vi "App.vi"() -> ()   [LabVIEW 2023]
uses:
  <vilib>/Instr/_visa.llb/VISA Configure Serial Port (Instr).vi
panel:
  out "Waveform Chart":dbl(graph)
  out "Temperatura Actual":string
  out "Temperatura":dbl(slide) scale=0.0..40.0
  in  "stop":bool
  in  "Puerto de comunicación":refnum<visa-resource-name>="COM3"
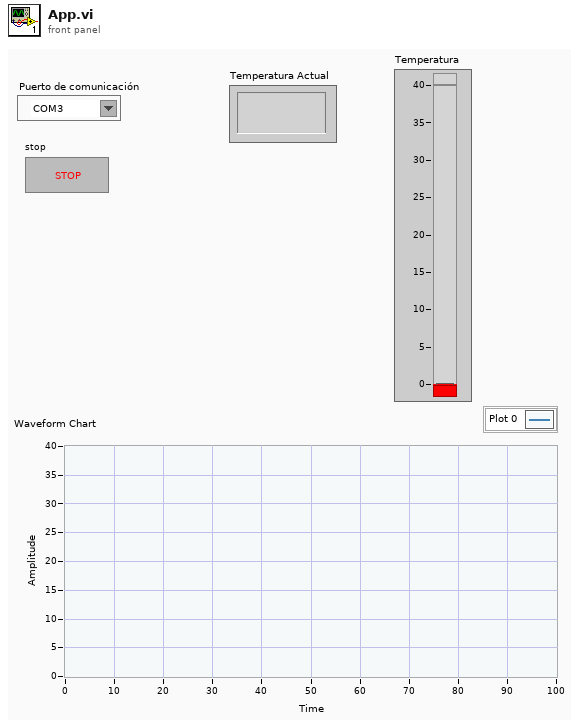
[diagram p1: front panel]
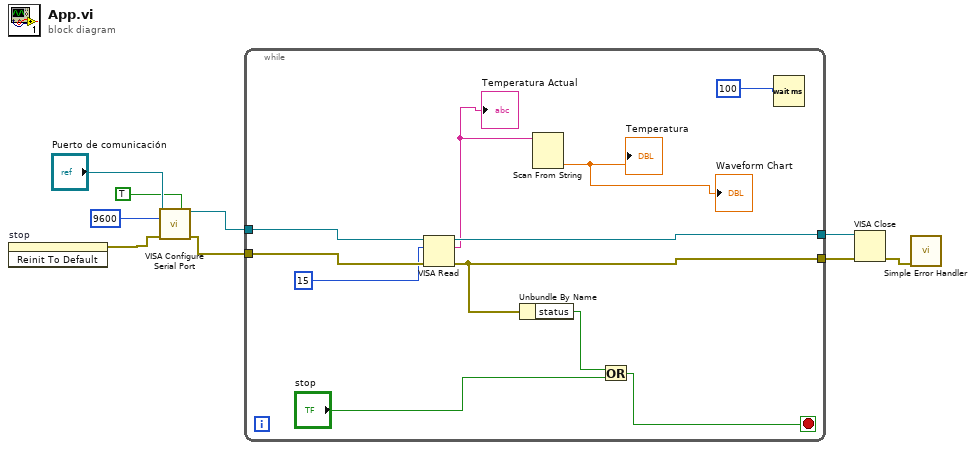
[diagram p0: block diagram]
diagram:
  n1 = invoke on="stop" class="Bool (strict)" method="Reinit To Default"() -> (error out=w1:errorcluster)  [unwired: 3 in, 2 out]
  n2 = call-poly "VISA Configure Serial Port"("VISA resource name"="Puerto de comunicación", "Enable Termination\nChar (T)"=TRUE ("Enable Termination\nChar (T)"), "baud rate (9600)"=u32 9600, "error in (no error)"=w1) -> ("VISA resource name out"=w6:refnum<visa-resource-name>, "error out"=w5:errorcluster)  [unwired: 10 in]
  n3 = while {
    tunnel: w6 -> [w20]
    tunnel: w5 -> [w19]
    tunnel: [w14] -> w3
    tunnel: [w13] -> w2
    stop <- w15 stop-if-true
    n4 = VISA Read(VISA resource name=w20, byte count=u32 15, error in (no error)=w19) -> (VISA resource name out=w14:refnum<visa-resource-name>, read buffer=w11:string, error out=w13:errorcluster)  [unwired: 1 out]
    "Temperatura Actual" <- w11
    n5 = Unbundle By Name(w13) -> ("status"=w17:bool)
    n6 = Scan From String(input string=w11) -> (output 1=→"Temperatura" →"Waveform Chart":dbl)  [unwired: 4 in, 3 out]
    n7 = Or(x=w17, y="stop") -> (x .or. y?=w15:bool)
    n8 = Wait (ms)(milliseconds to wait=u32 100) -> ()  [unwired: 1 out]
  }
  n9 = VISA Close(VISA resource name=w3, error in (no error)=w2) -> (error out=w4:errorcluster)
  n10 = call <vilib>:"Simple Error Handler.vi"("error in (no error)"=w4) -> ()  [unwired: 4 in, 5 out]
